vi "Obtain Priority Queue.vi"(8 "error in (no error)":errorcluster) -> (0 "error out":errorcluster, 3 "Priority Queue":refnum<class "Message Priority Queue.lvclass">)   [LabVIEW 2013, in "Actor Framework.lvlib" / "Message Priority Queue.lvclass"]
uses:
  <vilib>/ActorFramework/Message Priority Queue/Message Priority Queue.lvclass
  <vilib>/ActorFramework/Message Priority Queue/DVR Contents.ctl
  <vilib>/ActorFramework/Message/Message.lvclass
  <vilib>/ActorFramework/Message Priority Queue/Message Priority Queue.lvclass/Message Priority Queue.ctl
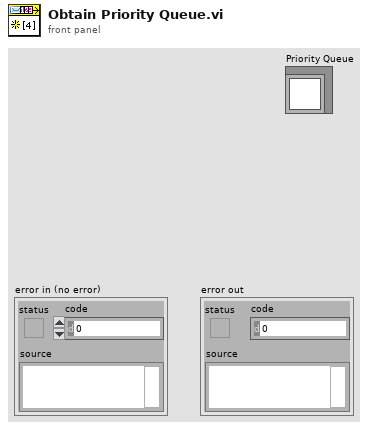
[diagram p1: front panel]
types:
  T1 = typedef "Actor Framework.lvlib/Message Priority Queue.lvclass/DVR Contents.ctl" = cluster{"# Waiting":u32, "Buffers":refnum<queue>[], "Wait Msg":refnum<queue>, "Wait Prior":refnum<queue>}
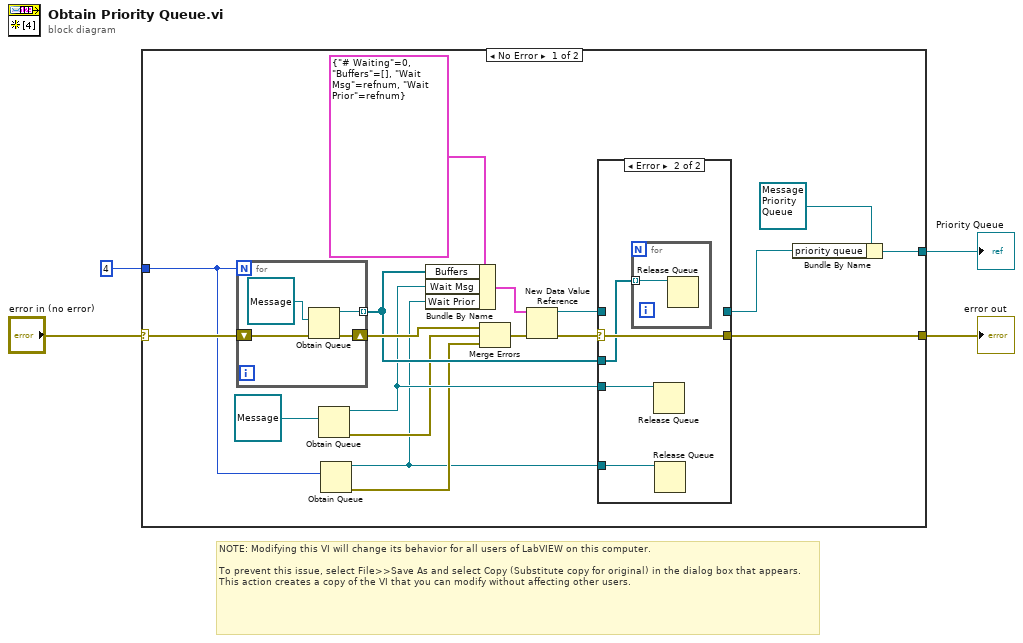
[diagram p0: block diagram]
diagram:
  # "NOTE: Modifying this VI will change its behavior for all users of LabVIEW on this computer.\n\nTo prevent this issue, select File>>Save As and select Copy (Substitute copy for original) in the dialog box that appears. This action creates a copy of the VI that you can modify without affecting other users."
  n1 = case shown="No Error" "error in (no error)" {
    selector: "error in (no error)" -> [w20 w34]
    tunnel: [w22 w34] -> w4
    tunnel: [w21 _] -> w3
    tunnel: 4 ("# of priorities") -> [w9 _]
    frame No Error {
      n2 = for {
        N: w9 -> [_]
        tunnel: [w33] -> w15 mode=indexing
        shift-right: [w32] -> w19
        shift-left: w20 -> [w31]
        n3 = Obtain Queue(element data type=refnum<class "Message.lvclass"> refnum ("Message"), error in (no error)=w31) -> (queue out=w33:refnum<queue>, error out=w32:errorcluster)  [unwired: 3 in, 1 out]
      }
      n4 = Obtain Queue(element data type=refnum<class "Message.lvclass"> refnum ("Message")) -> (queue out=w10:refnum<queue>, error out=w7:errorcluster)  [unwired: 4 in, 1 out]
      n5 = Obtain Queue(element data type=w9) -> (queue out=w5:refnum<queue>, error out=w6:errorcluster)  [unwired: 4 in, 1 out]
      n6 = Bundle By Name(cluster=T1 {"# Waiting"=0, "Buffers"=[], "Wait Msg"=refnum, "Wait Prior"=refnum} ("Priority Queue Internals"), "Buffers"=w15, "Wait Msg"=w10, "Wait Prior"=w5) -> (w16:T1)
      n7 = Merge Errors(w19, w7, w6) -> (w8:errorcluster)
      n8 = New Data Value Reference(data value=w16, error in=w8) -> (data value reference=w17:refnum<data-value>, error out=w18:errorcluster)
      n9 = case shown="Error" w18 {
        selector: w18 -> [w23 w28]
        tunnel: w17 -> [w24 _]
        tunnel: [w24 _] -> w13
        tunnel: [w23 w28] -> w22
        tunnel: w15 -> [_ w27]
        tunnel: w10 -> [_ w26]
        tunnel: w5 -> [_ w25]
        frame No Error {
        }
        frame Error {
          n10 = for {
            tunnel: w27 -> [w29] mode=indexing
            n11 = Release Queue(queue=w29) -> ()  [unwired: 2 in, 3 out]
          }
          n12 = Release Queue(queue=w26) -> ()  [unwired: 2 in, 3 out]
          n13 = Release Queue(queue=w25) -> ()  [unwired: 2 in, 3 out]
        }
      }
      n14 = Bundle By Name(cluster=refnum<class "Message Priority Queue.lvclass"> refnum ("Priority Queue.lvclass"), "priority queue"=w13) -> (w21:refnum<class "Message Priority Queue.lvclass">)
    }
    frame Error {
    }
  }
  "error out" <- w4
  "Priority Queue" <- w3
